vi "day 5 task 2.vi"() -> ()   [LabVIEW 2019]
panel:
  out "top of each stack":string
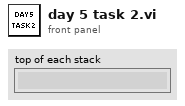
[diagram p1: front panel]
types:
  T1 = cluster{"no. crates to move":i32, "source col index":i32, "destination col index":i32}
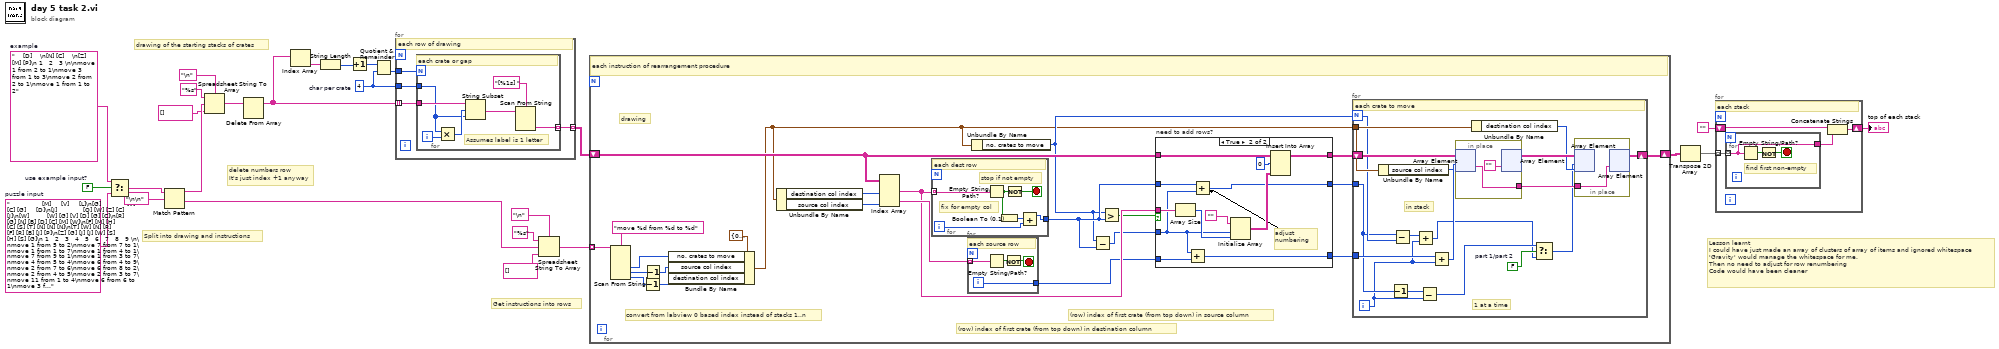
[diagram p0: block diagram]
diagram:
  w11 = 4  # char per crate
  w21 = FALSE  # use example input?
  w22 = "                [M]     [V]     [L]\n[G]             [V] [C] [G]     [D]\n[J]             [Q] [W] [Z] [C] [J]\n[W]         [W] [G] [V] [D] [G] [C]\n[R]     [G] [N] [B] [D] [C] [M] [W]\n[F] [M] [H] [C] [S] [T] [N] [N] [N]\n[T] [W] [N] [R] [F] [R] [B] [J] [P]\n[Z] [G] [J] [J] [W] [S] [H] [S] [G]\n 1   2   3   4   5   6   7   8   9 \n\nmove 1 from 5 to 2\nmove 7 from 7 to 1\nmove 1 from 1 to 7\nmove 1 from 4 to 1\nmove 7 from 9 to 1\nmove 1 from 3 to 7\nmove 4 from 5 to 4\nmove 6 from 4 to 9\nmove 2 from 7 to 6\nmove 6 from 8 to 2\nmove 2 from 4 to 5\nmove 2 from 3 to 7\nmove 11 from 1 to 4\nmove 6 from 6 to 1\nmove 3 from 5 to 3\nmove 5 from 9 to 8\nmove 1 from 2 to 3\nmove 2 from 7 to 9\nmove 7 from 1 to 2\nmove 1 from 5 to 3\nmove 1 from 5 to 3\nmove 5 from 8 to 5\nmove 3 from 5 to 4\nmove 1 from 1 to 7\nmove 1 from 3 to 8\nmove 2 from 6 to 3\nmove 3 from 3 to 4\nmove 1 from 6 to 2\nmove 5 from 4 to 2\nmove 2 from 5 to 3\nmove 2 from 7 to 1\nmove 1 from 8 to 1\nmove 7 from 1 to 7\nmove 4 from 4 to 2\nmove 7 from 4 to 1\nmove 10 from 1 to 5\nmove 10 from 5 to 2\nmove 11 from 2 to 3\nmove 1 from 1 to 6\nmove 1 from 4 to 7\nmove 4 from 7 to 1\nmove 6 from 2 to 5\nmove 2 from 1 to 3\nmove 1 from 9 to 5\nmove 2 from 9 to 6\nmove 1 from 6 to 1\nmove 3 from 5 to 4\nmove 20 from 3 to 9\nmove 3 from 7 to 1\nmove 3 from 5 to 2\nmove 3 from 4 to 8\nmove 3 from 1 to 3\nmove 3 from 1 to 2\nmove 2 from 6 to 1\nmove 10 from 9 to 6\nmove 6 from 6 to 7\nmove 4 from 6 to 3\nmove 11 from 2 to 6\nmove 1 from 8 to 9\nmove 13 from 2 to 3\nmove 1 from 1 to 9\nmove 1 from 9 to 4\nmove 1 from 8 to 2\nmove 1 from 8 to 2\nmove 4 from 7 to 8\nmove 8 from 6 to 9\nmove 3 from 2 to 3\nmove 3 from 8 to 4\nmove 11 from 9 to 2\nmove 7 from 9 to 6\nmove 1 from 1 to 5\nmove 4 from 4 to 9\nmove 21 from 3 to 1\nmove 1 from 3 to 9\nmove 7 from 6 to 3\nmove 6 from 1 to 2\nmove 13 from 1 to 5\nmove 2 from 1 to 2\nmove 3 from 9 to 3\nmove 2 from 2 to 3\nmove 2 from 6 to 4\nmove 3 from 3 to 5\nmove 13 from 5 to 2\nmove 5 from 3 to 4\nmove 2 from 7 to 9\nmove 2 from 4 to 2\nmove 1 from 3 to 8\nmove 1 from 6 to 1\nmove 4 from 3 to 7\nmove 2 from 5 to 7\nmove 1 from 7 to 2\nmove 1 from 5 to 9\nmove 4 from 7 to 8\nmove 1 from 1 to 9\nmove 6 from 8 to 1\nmove 4 from 4 to 8\nmove 25 from 2 to 9\nmove 1 from 4 to 3\nmove 1 from 3 to 7\nmove 4 from 8 to 1\nmove 1 from 7 to 4\nmove 3 from 1 to 6\nmove 5 from 2 to 1\nmove 1 from 5 to 1\nmove 1 from 4 to 1\nmove 24 from 9 to 6\nmove 9 from 1 to 6\nmove 1 from 5 to 6\nmove 1 from 1 to 9\nmove 1 from 2 to 8\nmove 1 from 8 to 1\nmove 3 from 1 to 8\nmove 36 from 6 to 3\nmove 2 from 7 to 3\nmove 1 from 2 to 5\nmove 1 from 5 to 2\nmove 1 from 6 to 2\nmove 10 from 3 to 2\nmove 3 from 8 to 2\nmove 1 from 1 to 7\nmove 2 from 2 to 6\nmove 10 from 9 to 1\nmove 2 from 6 to 4\nmove 13 from 3 to 4\nmove 8 from 3 to 7\nmove 8 from 1 to 2\nmove 5 from 3 to 8\nmove 3 from 1 to 9\nmove 1 from 7 to 1\nmove 7 from 4 to 5\nmove 1 from 1 to 2\nmove 14 from 2 to 6\nmove 2 from 7 to 2\nmove 8 from 4 to 8\nmove 3 from 7 to 9\nmove 2 from 9 to 8\nmove 2 from 7 to 1\nmove 1 from 7 to 8\nmove 1 from 6 to 8\nmove 1 from 9 to 3\nmove 4 from 2 to 7\nmove 6 from 6 to 1\nmove 3 from 1 to 9\nmove 1 from 1 to 7\nmove 6 from 5 to 6\nmove 1 from 5 to 2\nmove 1 from 6 to 8\nmove 5 from 7 to 5\nmove 1 from 2 to 9\nmove 2 from 3 to 4\nmove 9 from 8 to 4\nmove 8 from 4 to 8\nmove 6 from 6 to 7\nmove 5 from 6 to 4\nmove 7 from 9 to 7\nmove 7 from 8 to 7\nmove 5 from 8 to 4\nmove 3 from 1 to 6\nmove 1 from 2 to 7\nmove 1 from 1 to 4\nmove 4 from 5 to 2\nmove 2 from 6 to 9\nmove 1 from 3 to 7\nmove 1 from 5 to 1\nmove 1 from 8 to 9\nmove 1 from 6 to 1\nmove 1 from 2 to 7\nmove 2 from 8 to 1\nmove 2 from 1 to 8\nmove 3 from 2 to 4\nmove 1 from 6 to 1\nmove 17 from 4 to 1\nmove 3 from 2 to 7\nmove 13 from 7 to 8\nmove 1 from 2 to 6\nmove 14 from 1 to 4\nmove 2 from 8 to 5\nmove 1 from 9 to 7\nmove 2 from 5 to 4\nmove 1 from 9 to 3\nmove 5 from 1 to 5\nmove 3 from 4 to 1\nmove 1 from 3 to 2\nmove 7 from 4 to 5\nmove 9 from 7 to 8\nmove 5 from 4 to 2\nmove 1 from 1 to 3\nmove 1 from 9 to 2\nmove 15 from 8 to 6\nmove 1 from 3 to 7\nmove 11 from 6 to 5\nmove 1 from 4 to 8\nmove 3 from 1 to 7\nmove 5 from 7 to 5\nmove 27 from 5 to 1\nmove 8 from 8 to 4\nmove 1 from 2 to 6\nmove 3 from 6 to 1\nmove 9 from 1 to 5\nmove 5 from 5 to 7\nmove 2 from 2 to 1\nmove 2 from 5 to 4\nmove 6 from 7 to 6\nmove 1 from 5 to 2\nmove 1 from 7 to 8\nmove 4 from 6 to 8\nmove 5 from 6 to 3\nmove 1 from 7 to 1\nmove 5 from 4 to 3\nmove 6 from 8 to 2\nmove 1 from 7 to 8\nmove 2 from 8 to 9\nmove 10 from 3 to 5\nmove 9 from 5 to 2\nmove 3 from 4 to 8\nmove 1 from 5 to 7\nmove 2 from 9 to 7\nmove 2 from 8 to 3\nmove 1 from 3 to 8\nmove 19 from 1 to 7\nmove 4 from 2 to 7\nmove 2 from 4 to 3\nmove 3 from 3 to 2\nmove 2 from 8 to 3\nmove 2 from 5 to 8\nmove 1 from 2 to 3\nmove 2 from 8 to 3\nmove 5 from 2 to 5\nmove 9 from 7 to 5\nmove 13 from 5 to 9\nmove 7 from 2 to 6\nmove 2 from 6 to 9\nmove 1 from 2 to 1\nmove 5 from 6 to 7\nmove 1 from 5 to 7\nmove 6 from 1 to 2\nmove 5 from 3 to 6\nmove 6 from 7 to 2\nmove 3 from 6 to 4\nmove 3 from 7 to 4\nmove 12 from 7 to 6\nmove 5 from 4 to 1\nmove 2 from 7 to 4\nmove 3 from 4 to 6\nmove 16 from 6 to 3\nmove 4 from 1 to 4\nmove 1 from 1 to 9\nmove 3 from 9 to 2\nmove 1 from 4 to 6\nmove 9 from 3 to 7\nmove 2 from 6 to 3\nmove 3 from 3 to 9\nmove 15 from 2 to 7\nmove 19 from 7 to 4\nmove 15 from 9 to 2\nmove 16 from 2 to 8\nmove 6 from 3 to 5\nmove 4 from 7 to 5\nmove 15 from 8 to 7\nmove 19 from 4 to 2\nmove 1 from 8 to 3\nmove 16 from 2 to 1\nmove 9 from 7 to 6\nmove 7 from 2 to 8\nmove 2 from 2 to 7\nmove 1 from 9 to 5\nmove 1 from 3 to 4\nmove 6 from 1 to 2\nmove 8 from 5 to 1\nmove 1 from 5 to 1\nmove 18 from 1 to 8\nmove 7 from 7 to 5\nmove 7 from 5 to 3\nmove 4 from 3 to 6\nmove 13 from 8 to 5\nmove 12 from 8 to 1\nmove 5 from 1 to 6\nmove 15 from 5 to 4\nmove 1 from 1 to 6\nmove 12 from 6 to 3\nmove 8 from 3 to 4\nmove 2 from 7 to 3\nmove 9 from 3 to 1\nmove 5 from 2 to 9\nmove 16 from 4 to 3\nmove 10 from 1 to 3\nmove 2 from 1 to 5\nmove 1 from 3 to 1\nmove 5 from 6 to 1\nmove 4 from 9 to 3\nmove 1 from 2 to 8\nmove 1 from 8 to 1\nmove 1 from 9 to 8\nmove 2 from 5 to 9\nmove 9 from 4 to 1\nmove 3 from 1 to 3\nmove 2 from 6 to 8\nmove 3 from 8 to 5\nmove 2 from 1 to 5\nmove 2 from 9 to 8\nmove 1 from 8 to 6\nmove 2 from 5 to 3\nmove 19 from 3 to 1\nmove 2 from 4 to 2\nmove 1 from 5 to 6\nmove 2 from 2 to 3\nmove 1 from 8 to 6\nmove 8 from 3 to 9\nmove 6 from 3 to 7\nmove 2 from 6 to 2\nmove 1 from 6 to 1\nmove 1 from 1 to 8\nmove 1 from 8 to 9\nmove 1 from 7 to 3\nmove 19 from 1 to 5\nmove 21 from 5 to 2\nmove 13 from 2 to 6\nmove 13 from 1 to 8\nmove 7 from 9 to 7\nmove 2 from 9 to 2\nmove 10 from 8 to 3\nmove 1 from 1 to 6\nmove 10 from 2 to 4\nmove 11 from 3 to 5\nmove 8 from 5 to 6\nmove 1 from 3 to 7\nmove 2 from 8 to 6\nmove 2 from 2 to 8\nmove 3 from 7 to 6\nmove 2 from 8 to 6\nmove 1 from 1 to 2\nmove 24 from 6 to 5\nmove 2 from 3 to 8\nmove 1 from 8 to 6\nmove 7 from 7 to 9\nmove 4 from 6 to 9\nmove 1 from 8 to 9\nmove 21 from 5 to 9\nmove 2 from 7 to 2\nmove 1 from 8 to 5\nmove 1 from 7 to 3\nmove 12 from 9 to 6\nmove 6 from 6 to 3\nmove 12 from 9 to 4\nmove 4 from 5 to 6\nmove 13 from 4 to 2\nmove 8 from 4 to 8\nmove 10 from 6 to 8\nmove 11 from 8 to 9\nmove 4 from 8 to 4\nmove 2 from 4 to 3\nmove 8 from 3 to 8\nmove 2 from 6 to 8\nmove 1 from 3 to 8\nmove 6 from 2 to 4\nmove 1 from 4 to 8\nmove 1 from 9 to 7\nmove 13 from 8 to 4\nmove 1 from 7 to 1\nmove 1 from 1 to 4\nmove 8 from 4 to 7\nmove 3 from 5 to 7\nmove 19 from 9 to 7\nmove 3 from 2 to 7\nmove 1 from 8 to 2\nmove 13 from 7 to 6\nmove 1 from 2 to 4\nmove 4 from 6 to 2\nmove 1 from 8 to 3\nmove 7 from 6 to 8\nmove 1 from 6 to 2\nmove 1 from 2 to 7\nmove 9 from 2 to 3\nmove 1 from 6 to 2\nmove 21 from 7 to 5\nmove 9 from 5 to 3\nmove 19 from 3 to 9\nmove 5 from 8 to 5\nmove 2 from 2 to 1\nmove 2 from 1 to 8\nmove 6 from 4 to 5\nmove 3 from 8 to 7\nmove 15 from 9 to 2\nmove 2 from 2 to 5\nmove 3 from 9 to 6\nmove 5 from 4 to 5\nmove 11 from 2 to 6\nmove 1 from 8 to 6\nmove 1 from 9 to 5\nmove 1 from 7 to 3\nmove 6 from 5 to 6\nmove 1 from 4 to 6\nmove 1 from 3 to 4\nmove 13 from 5 to 2\nmove 16 from 6 to 9\nmove 4 from 4 to 5\nmove 2 from 6 to 2\nmove 2 from 6 to 4\nmove 2 from 4 to 5\nmove 2 from 7 to 8\nmove 2 from 6 to 3\nmove 2 from 5 to 8\nmove 14 from 5 to 7\nmove 4 from 8 to 1\nmove 4 from 1 to 6\nmove 1 from 3 to 9\nmove 1 from 6 to 1\nmove 2 from 7 to 3\nmove 2 from 3 to 7\nmove 2 from 5 to 2\nmove 9 from 9 to 2\nmove 13 from 7 to 3\nmove 12 from 3 to 9\nmove 2 from 6 to 8\nmove 14 from 2 to 9\nmove 2 from 8 to 9\nmove 10 from 2 to 1\nmove 1 from 7 to 4\nmove 2 from 3 to 8\nmove 4 from 2 to 1\nmove 1 from 8 to 3\nmove 1 from 2 to 6\nmove 1 from 8 to 3\nmove 4 from 9 to 4\nmove 1 from 3 to 5\nmove 1 from 5 to 1\nmove 1 from 3 to 9\nmove 12 from 1 to 8\nmove 10 from 8 to 5\nmove 7 from 5 to 6\nmove 1 from 1 to 9\nmove 3 from 5 to 1\nmove 1 from 1 to 3\nmove 16 from 9 to 7\nmove 4 from 4 to 3\nmove 1 from 4 to 9\nmove 15 from 7 to 8\nmove 15 from 9 to 1\nmove 8 from 1 to 6\nmove 1 from 9 to 3\nmove 17 from 6 to 2\nmove 1 from 9 to 1\nmove 15 from 2 to 7\nmove 14 from 8 to 9\nmove 12 from 7 to 9\nmove 12 from 9 to 3\nmove 3 from 7 to 9\nmove 1 from 7 to 4\nmove 7 from 9 to 6\nmove 1 from 4 to 6\nmove 11 from 9 to 6\nmove 2 from 1 to 2\nmove 18 from 6 to 4\nmove 4 from 2 to 7\nmove 2 from 7 to 3\nmove 2 from 7 to 8\nmove 4 from 1 to 5\nmove 1 from 9 to 2\nmove 2 from 5 to 4\nmove 5 from 1 to 3\nmove 2 from 3 to 7\nmove 2 from 3 to 9\nmove 1 from 6 to 7\nmove 1 from 2 to 9\nmove 2 from 8 to 1\nmove 3 from 1 to 3\nmove 2 from 5 to 8\nmove 2 from 3 to 5\nmove 1 from 5 to 2\nmove 1 from 1 to 3\nmove 1 from 9 to 2\nmove 1 from 9 to 1\nmove 3 from 7 to 6\nmove 1 from 1 to 9\nmove 2 from 8 to 9\nmove 1 from 2 to 3\nmove 2 from 8 to 2\nmove 2 from 6 to 5\nmove 1 from 8 to 5\nmove 3 from 2 to 5\nmove 3 from 4 to 8\nmove 1 from 8 to 2\nmove 3 from 9 to 7\nmove 3 from 7 to 1\nmove 1 from 9 to 6\nmove 3 from 1 to 2\nmove 2 from 8 to 7\nmove 2 from 7 to 9\nmove 2 from 6 to 5\nmove 3 from 5 to 3\nmove 1 from 2 to 5\nmove 3 from 2 to 7\nmove 2 from 5 to 6\nmove 15 from 4 to 9\nmove 1 from 3 to 1\nmove 25 from 3 to 4\nmove 3 from 7 to 3\nmove 5 from 9 to 5\nmove 10 from 9 to 5\nmove 9 from 5 to 1\nmove 5 from 5 to 2\nmove 1 from 6 to 7\nmove 5 from 5 to 8"  # puzzle input
  w23 = "    [D]    \n[N] [C]    \n[Z] [M] [P]\n 1   2   3 \n\nmove 1 from 2 to 1\nmove 3 from 1 to 3\nmove 2 from 2 to 1\nmove 1 from 1 to 2"  # example
  # "Lesson learnt\nI could have just made an array of clusters of array of items and ignored whitespace\n'Gravity' would manage the whitespace for me.\nThen no need to adjust for row renumbering\nCode would have been cleaner"
  # "Split into drawing and instructions"
  # "Get instructions into rows"
  # "delete numbers row\nIt's just index +1 anyway"
  # "drawing of the starting stacks of crates"
  n1 = Select(t=w23, s=w21, f=w22) -> (s? t:f=w19:string)
  n2 = Match Pattern(string=w19, regular expression="\n\n" ("example")) -> (before substring=w14:string, after substring=w17:string)  [unwired: 1 in, 2 out]
  n3 = Spreadsheet String To Array(delimiter (Tab)="\n", format string="%s", spreadsheet string=w14, array type (2D Dbl)=string[] []) -> (array=w9:string[])
  n4 = Delete From Array(array=w9) -> (array with subset deleted=w10:string[])  [unwired: 2 in, 1 out]
  n5 = Index Array(array=w10) -> (element=w13:string)  [unwired: 1 in]
  n6 = String Length(string=w13) -> (length=w1:i32)
  n7 = Increment(x=w1) -> (x+1=w2:i32)
  n8 = Quotient & Remainder(x=w2, y=w11) -> (floor(x/y)=w3:i32)  [unwired: 1 out]
  n9 = for {
    tunnel: w10 -> [w27] mode=indexing
    tunnel: w11 -> [w29]
    tunnel: [w30] -> w8 mode=indexing
    tunnel: w3 -> [w28]
    # "each row of drawing"
    n10 = for {
      N: w28 -> [_]
      tunnel: w29 -> [w31]
      tunnel: w27 -> [w37]
      tunnel: [w32] -> w30 mode=indexing
      i -> [w35]
      # "Assumes label is 1 letter"
      # "each crate or gap"
      n11 = Multiply(x=w31, y=w35) -> (x*y=w36:i32)
      n12 = String Subset(string=w37, offset (0)=w36, length (rest)=w31) -> (substring=w33:string)
      n13 = Scan From String(format string="[%1s] ", input string=w33) -> (output 1=w32:string)  [unwired: 3 in, 3 out]
    }
  }
  n14 = Spreadsheet String To Array(delimiter (Tab)="\n", format string="%s", spreadsheet string=w17, array type (2D Dbl)=string[] []) -> (array=w20:string[])
  n15 = for {
    tunnel: w20 -> [w60] mode=indexing
    shift-right: [w51] -> w7
    shift-left: w8 -> [w52]
    # "drawing"
    # "(row) index of first crate (from top down) in source column"
    # "(row) index of first crate (from top down) in destination column"
    # "convert from labview 0 based index instead of stacks 1..n"
    # "each instruction of rearrangement procedure"
    n16 = Scan From String(format string="move %d from %d to %d", input string=w60) -> (output 1=w55:i32, output 2=w58:i32, output 3=w57:i32)  [unwired: 5 in, 3 out]
    n17 = Decrement(x=w57) -> (x-1=w53:i32)
    n18 = Decrement(x=w58) -> (x-1=w54:i32)
    n19 = Bundle By Name(cluster=T1 {"no. crates to move"=0, "source col index"=0, "destination col index"=0}, "no. crates to move"=w55, "source col index"=w54, "destination col index"=w53) -> (w38:T1)
    n20 = Unbundle By Name(w38) -> ("destination col index"=w49:i32, "source col index"=w50:i32)
    n21 = Index Array(array=w52, index (col) #1=w49, index (col) #2=w50) -> (element #1=w47:string[], element #2=w48:string[])  [unwired: 2 in]
    n22 = for {
      tunnel: [w101] -> w45
      tunnel: w47 -> [w106] mode=indexing
      i -> [w103]
      stop <- w105 stop-if-true
      # "fix for empty col"
      # "stop if not empty"
      # "each dest row"
      n23 = Empty String/Path?(string/path=w106) -> (empty?=w102:bool)
      n24 = Boolean To (0,1)(Boolean=w102) -> (0, 1=w104:i16)
      n25 = Not(x=w102) -> (.not. x?=w105:bool)
      n26 = Add(x=w104, y=w103) -> (x+y=w101:i32)
    }
    n27 = for {
      tunnel: [w100] -> w44
      tunnel: w48 -> [w99] mode=indexing
      i -> [w100]
      stop <- w98 stop-if-true
      # "each source row"
      n28 = Empty String/Path?(string/path=w99) -> (empty?=w97:bool)
      n29 = Not(x=w97) -> (.not. x?=w98:bool)
    }
    n30 = Unbundle By Name(w38) -> ("no. crates to move"=w43:i32)
    n31 = Subtract(x=w43, y=w45) -> (x-y=w46:i32)
    n32 = Greater?(x=w43, y=w45) -> (0:w41:bool)
    n33 = case "need to add rows?" shown="True" w41 {
      tunnel: w47 -> [_ w96]
      tunnel: w46 -> [_ w87]
      tunnel: w52 -> [w82 w91]
      tunnel: [w82 w90] -> w42
      tunnel: [w84 w85] -> w39
      tunnel: w45 -> [w84 w89]
      tunnel: [w83 w86] -> w40
      tunnel: w44 -> [w83 w88]
      frame False {
      }
      frame True {
        # "adjust numbering"
        n34 = Array Size(array=w96) -> (size(s)=w94:i32)
        n35 = Add(x=w87, y=w88) -> (x+y=w86:i32)
        n36 = Add(x=w89, y=w87) -> (x+y=w85:i32)
        n37 = Initialize Array("", w87, w94) -> (w92:string[][])
        n38 = Insert Into Array(array=w91, index (row)=0, new element=w92) -> (w90:string[][])  [unwired: 1 in]
      }
    }
    n39 = for {
      N: w43 -> [w69]
      tunnel: w40 -> [w76]
      tunnel: w39 -> [w68]
      tunnel: w38 -> [w73]
      shift-right: [w70] -> w51
      shift-left: w42 -> [w78]
      i -> [w67]
      w65 = FALSE  # part 1/part 2
      # "in stack"
      # "1 at a time"
      # "each crate to move"
      n40 = Unbundle By Name(w73) -> ("source col index"=w74:i32)
      n41 = Decrement(x=w68) -> (x-1=w63:i32)
      n42 = Subtract(x=w68, y=w69) -> (x-y=w66:i32)
      n43 = Add(x=w66, y=w67) -> (x+y=w62:i32)
      n44 = Subtract(x=w63, y=w67) -> (x-y=w64:i32)
      n45 = Add(x=w76, y=w67) -> (x+y=w75:i32)
      n46 = in-place {
        in-place-border: [w81] -> w71
        n47 = in-place-array #1(w78, w75, w74) -> (w81:string)
        n48 = in-place-array #1("") -> (w77:string[][])  [unwired: 2 out]
      }
      n49 = Unbundle By Name(w73) -> ("destination col index"=w72:i32)
      n50 = Select(t=w64, s=w65, f=w62) -> (s? t:f=w61:i32)
      n51 = in-place {
        in-place-border: w71 -> [w79]
        n52 = in-place-array #2(w77, w61, w72) -> ()  [unwired: 1 out]
        n53 = in-place-array #2(w79) -> (w70:string[][])  [unwired: 2 out]
      }
    }
  }
  n54 = Transpose 2D Array(2D array=w7) -> (transposed array=w6:string[][])
  n55 = for {
    tunnel: w6 -> [w110] mode=indexing
    shift-right: [w109] -> w4
    shift-left: "" -> [w108]
    # "each stack"
    n56 = for {
      tunnel: w110 -> [w111] mode=indexing
      tunnel: [w111] -> w107
      stop <- w112 stop-if-true
      # "find first non-empty"
      n57 = Empty String/Path?(string/path=w111) -> (empty?=w113:bool)
      n58 = Not(x=w113) -> (.not. x?=w112:bool)
    }
    n59 = Concatenate Strings(w108, w107) -> (w109:string)
  }
  "top of each stack" <- w4
